vi "getStopMechanism.vi"(8 "error in (no error)":errorcluster, 11 "ExampleTask_MsgUserEventStopNotifier In":refnum<class "Task_MsgUserEventStopMech.lvclass">) -> (0 "error out":errorcluster, 2 "stopMechanism":refnum<class "ITaskStopMechanism.lvclass">, 3 "ExampleTask_MsgUserEventStopNotifier Out":refnum<class "Task_MsgUserEventStopMech.lvclass">)   [LabVIEW 2023, in "Task_MsgUserEventStopMech.lvclass"]
doc: "Returns the stop mechanism type used by the task."
uses:
  Task_MsgUserEventStopMech.lvclass
  MsgUserEventStopMech/MsgUserEventStopMechanism.lvclass
  ITaskStopMechanism/ITaskStopMechanism.lvclass
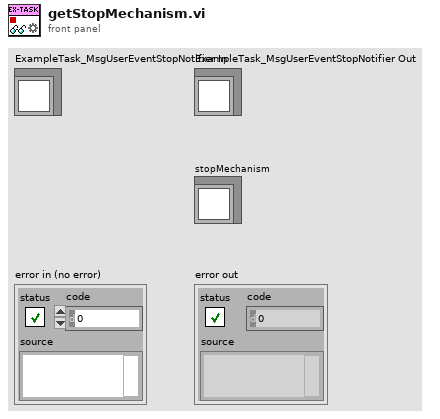
[diagram p1: front panel]
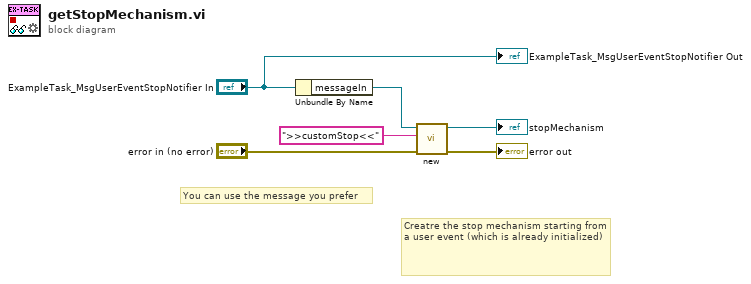
[diagram p0: block diagram]
diagram:
  # "You can use the message you prefer"
  # "Creatre the stop mechanism starting from a user event (which is already initialized)"
  n1 = Unbundle By Name("ExampleTask_MsgUserEventStopNotifier In") -> ("messageIn"=w5:refnum<user-event>)
  n2 = call "new.vi"("error in (no error)"="error in (no error)", "stopMessage"=">>customStop<<", "msgUserEvent"=w5) -> ("error out"=→"error out":errorcluster, "MsgUserEventStopMechanism Out"=→"stopMechanism":refnum<class "MsgUserEventStopMechanism.lvclass">)  [unwired: 7 in]
  "ExampleTask_MsgUserEventStopNotifier Out" <- "ExampleTask_MsgUserEventStopNotifier In"
